vi "SL TAGS Update Class Values From Server.vi"(8 "error in (no error)":errorcluster, 10 "Tag Type":T1, 11 "EEISysLink in":refnum<class "EEISysLink.lvclass">) -> (0 "error out":errorcluster, 3 "EEISysLink out":refnum<class "EEISysLink.lvclass">)   [LabVIEW 2017, in "EEISysLink.lvclass"]
doc: "Will return the current value of all selected tag types. Will retrieve the values within the selected scope as follows. \n\nServer = Get updated values from the SystemLink server, update the class tag values, and return them.\nLocal = Return the values of the class tags\n\nJames Tillett P.E.\nEndeavor Engineering Inc.\nwww.endeavoreng.com"
uses:
  EEISysLink.lvclass
  Controls/SL Tag Type.ctl
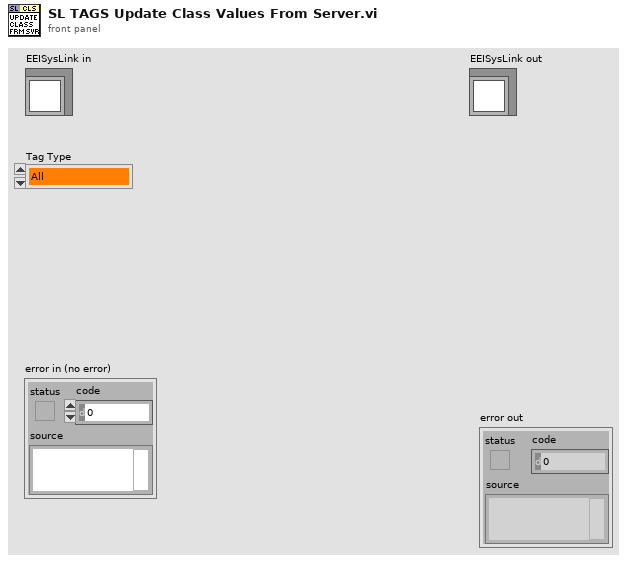
[diagram p1: front panel]
types:
  T1 = typedef "EEISysLink.lvclass/SL Tag Type.ctl" = enum16{"All", "Supervisor", "Worker"}
  T2 = typedef "EEISysLink.lvclass/SL Tag.ctl" = cluster{"Class Properties":T3, "SL Tag":refnum<class "NI Skyline Tag.lvclass">, "SystemLink Cluster":T7, "Class Value":variant}
  T3 = typedef "EEISysLink.lvclass/SL Tag Properties.ctl" = cluster{"Class Data Type":T4, "Name":string, "Description":string, "Interpolation Method":T5, "Unit of Measure":T6, "Maximum Interpolation":string, "Role":T1}
  T4 = typedef "EEISysLink.lvclass/SL Tag Data Type.ctl" = enum16{"Double", "Integer", "String", "Boolean", "Waveform"}
  T5 = typedef "EEISysLink.lvclass/SL Tag Interpolation Method.ctl" = enum16{"linear", "pilinear", "step"}
  T6 = typedef "EEISysLink.lvclass/SL Tag Unit of Measure.ctl" = enum16{"no units", "Second", "Hour", "Minute", "Day", "Year", "Month", "Week", "Foot", "Yard", "Meter", "Centimeter", "Inch", "Mile", "Nautical Mile", "Miles per Hour", "Meters per second", "Square meter", "Cubic meter", "Cubic centimeter", "Cubic inch", "Liter", "Gallon", "Gallons dry US", "Gallon UK", "Percent", "Revolutions per minute", "Revolution", "Degree angle", "Astronomical Unit", "Atom", "Atomic mass", "Bar", "Byte", "C (speed of light)", "Curie", "Decibel", "Electron Volt", "Ounce", "Knot", "G", "Grade", "Are", "Hectare", "Faraday", "Franklin", "Gilbert", "Erg", "Lambert", "Maxwell", "Gauss", "Electron mass", "Kilogram force", "Pound force", "Rad", "Centiradian", "Sphere", "Mach", "Fluid Ounces", "Fluid Ounces UK", "Fahrenheit", "Celsius", "Kelvin", "Rankine", "Gram", "Kilogram", "Pound", "Short/US Ton", "Long/UK ton", "Metric ton", "Mole", "Pounds per square inch", "Inches water column", "Torr", "Millitorr", "Millimeter mercury", "Inches mercury", "Bar (2)", "Atmosphere", "Pascal", "Watt", "kiloWatt", "Horsepower", "Kilowatt Hour", "British thermal units", "Millions of BTU", "Ampere", "Candela", "Radian", "Steradian", "Bit", "Hertz", "Newton", "Joule", "Coulomb", "Volt", "Farad", "Ohm", "Siemens", "Weber", "Tesla", "Henry", "Lumen", "Lux", "Becqueral", "Gray", "Sievert", "Katal", "Angstrom", "Light Year", "Parsec", "Point", "Pixel", "Dyne", "Kilogram force (2)", "Pound force (2)", "Rem", "Rutherford", "Roentgen"}
  T7 = typedef "NI Skyline Tag.lvlib/Tag Cluster.ctl" = cluster{"Path":string, "Data Type":T8, "Value":variant, "Time Stamp":timestamp}
  T8 = typedef "NI Skyline Tag.lvlib/DataType.ctl" = enum32{"Double", "Integer", "String"}
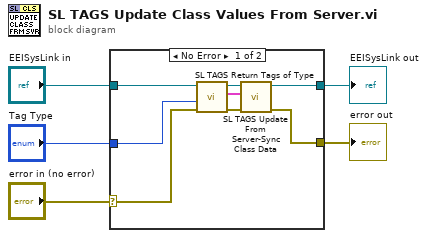
[diagram p0: block diagram]
diagram:
  n1 = case shown="No Error" "error in (no error)" {
    selector: "error in (no error)" -> [w11 w15]
    tunnel: [w8 w15] -> w4
    tunnel: [w9 w14] -> w2
    tunnel: "EEISysLink in" -> [w13 w14]
    tunnel: "Tag Type" -> [w12 _]
    frame No Error {
      n2 = call "SL TAGS Return Tags of Type.vi"("error in (no error)"=w11, "Tag Type"=w12, "EEISysLink in"=w13) -> ("error out"=w6:errorcluster, "Tags of Type"=w7:T2[], "EEISysLink out"=w10:refnum<class "EEISysLink.lvclass">)  [unwired: 6 in]
      n3 = call "SL TAGS Update From Server-Sync Class Data.vi"("error in (no error)"=w6, "Tags to Update"=w7, "EEISysLink in"=w10) -> ("error out"=w8:errorcluster, "EEISysLink out"=w9:refnum<class "EEISysLink.lvclass">)  [unwired: 6 in, 1 out]
    }
    frame Error {
    }
  }
  "error out" <- w4
  "EEISysLink out" <- w2
